vi "SERIAL_GetAngle.vi"(11 "navX DevRef":T1={"SerialPortRef"={"DevStatus"={"status"=FALSE, "code"=0, "source"=""}, "Serial Port Name"=""}, "Board Information"={"WhoAmI (50 | 0x32)"=0, "Board Revision"=0, "Firmware Major Version"=0, "Firmware Minor Version"=0, "NAVX_BOARD_CAPABILITY"={"OMNIMOUNT"=FALSE, "YAW_RESET"=FALSE, "VEL_AND_DISP"=FALSE}, "NAVX_BOARD_YAW_AXIS"={"BOARD_YAW_AXIS_UP"=FALSE, "BOARD_YAW_AXIS"=0}}, "Status"={"Update Rate Hz"=0, "Accelerometer Full-Scale Range"=0, "Gyro Full-Scale Range"=0, "NAVX_OP_STATUS"=0, "NAVX_CAL_STATUS"=0, "NAVX_SELFTEST_STATUS"=0, "NAVX_SENSOR_STATUS"={"MOVING"=FALSE, "YAW_STABLE"=FALSE, "MAG_DISTURBANCE"=FALSE, "ALTITUDE_VALID"=FALSE, "SEALEVEL_PRESS_SET"=FALSE, "FUSED_HEADING_VALID"=FALSE}}, "Offsets"={"Yaw"=50.0, "Quat W"=0.0, "Quat X"=0.0, "Quat Y"=0.0, "Quat Z"=0.0}, "Update Rate (4Hz-60Hz)"=50, "Nav6Mode (YPR)"=enum."RawSensorData", "refnum name"="", "error"={"status"=FALSE, "code"=0, "source"=""}, "Loop VI Refnum"=refnum, "Serial Port"=enum."Onboard RS-232"} {"Status"."NAVX_OP_STATUS" items=["INITIALIZING", "SELFTEST_IN_PROGRESS", "ERROR", "IMU_AUTOCAL_IN_PROGRESS", "NORMAL"]; "Status"."NAVX_CAL_STATUS" items=["IMU_CAL_STATE_MASK"=3, "IMU_CAL_INPROGRESS"=0, "IMU_CAL_ACCUMULATE"=1, "IMU_CAL_COMPLETE"=2, "MAG_CAL_COMPLETE"=4, "BARO_CAL_COMPLETE"=8]}) -> (1 "Valid?":bool, 2 "ContinuousAngle":dbl, 3 "navX DevRef 2":T1={"SerialPortRef"={"DevStatus"={"status"=FALSE, "code"=0, "source"=""}, "Serial Port Name"=""}, "Board Information"={"WhoAmI (50 | 0x32)"=0, "Board Revision"=0, "Firmware Major Version"=0, "Firmware Minor Version"=0, "NAVX_BOARD_CAPABILITY"={"OMNIMOUNT"=FALSE, "YAW_RESET"=FALSE, "VEL_AND_DISP"=FALSE}, "NAVX_BOARD_YAW_AXIS"={"BOARD_YAW_AXIS_UP"=FALSE, "BOARD_YAW_AXIS"=0}}, "Status"={"Update Rate Hz"=0, "Accelerometer Full-Scale Range"=0, "Gyro Full-Scale Range"=0, "NAVX_OP_STATUS"=0, "NAVX_CAL_STATUS"=0, "NAVX_SELFTEST_STATUS"=0, "NAVX_SENSOR_STATUS"={"MOVING"=FALSE, "YAW_STABLE"=FALSE, "MAG_DISTURBANCE"=FALSE, "ALTITUDE_VALID"=FALSE, "SEALEVEL_PRESS_SET"=FALSE, "FUSED_HEADING_VALID"=FALSE}}, "Offsets"={"Yaw"=50.0, "Quat W"=0.0, "Quat X"=0.0, "Quat Y"=0.0, "Quat Z"=0.0}, "Update Rate (4Hz-60Hz)"=50, "Nav6Mode (YPR)"=enum."RawSensorData", "refnum name"="", "error"={"status"=FALSE, "code"=0, "source"=""}, "Loop VI Refnum"=refnum, "Serial Port"=enum."Onboard RS-232"} {"Status"."NAVX_OP_STATUS" items=["INITIALIZING", "SELFTEST_IN_PROGRESS", "ERROR", "IMU_AUTOCAL_IN_PROGRESS", "NORMAL"]; "Status"."NAVX_CAL_STATUS" items=["IMU_CAL_STATE_MASK"=3, "IMU_CAL_INPROGRESS"=0, "IMU_CAL_ACCUMULATE"=1, "IMU_CAL_COMPLETE"=2, "MAG_CAL_COMPLETE"=4, "BARO_CAL_COMPLETE"=8]})   [LabVIEW 2014, in "navX-MXP IMU.lvlib"]
doc: "Returns the angle, in degrees, from the original heading that the robot is currently facing.\n\nNote that this angle is continuous (meaning that it can return values greater than 360 degrees and less than -360 degrees. You can device by 360 and use the remainder to yield and angle with a value from -360 to 360 degrees.\n\nThis VI is created to provide an interface which is compatible with the WPI LabVIEW Library GetAngle.vi ."
uses:
  navX-MXP IMU.lvlib
  TypeDefs/navX Serial DevRef.ctl
  <vilib>/Rock Robotics/WPI/SerialPort/WPI_SerialPortRef.ctl
  COMMON/TypeDefs/Data TypeDefs/navX Board Information.ctl
  COMMON/TypeDefs/Value TypeDefs/navX NAVX_BOARD_CAPABILITY.ctl
  COMMON/TypeDefs/Value TypeDefs/navX NAVX_BOARD_YAW_AXIS.ctl
  COMMON/TypeDefs/Data TypeDefs/navX Status Data.ctl
  COMMON/TypeDefs/Value TypeDefs/navX NAVX_OP_STATUS.ctl
  COMMON/TypeDefs/Value TypeDefs/navX NAVX_CAL_STATUS.ctl
  COMMON/TypeDefs/Value TypeDefs/navX NAVX_SENSOR_STATUS.ctl
  TypeDefs/navX Serial Mode.ctl
  IO/NI WPI/WPI_SerialPort_USB.ctl
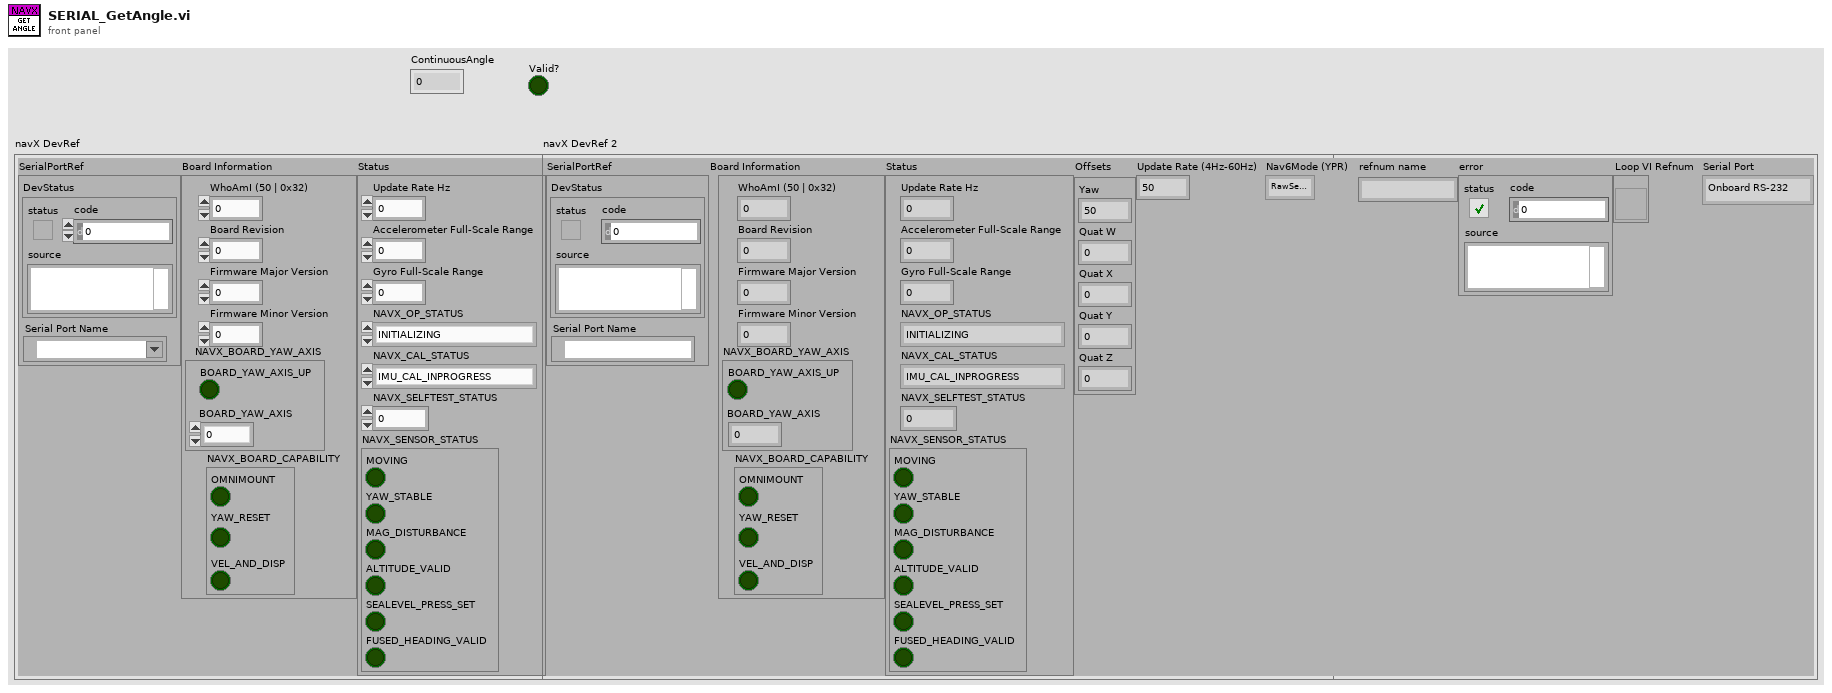
[diagram p1: front panel]
types:
  T1 = typedef "navX-MXP IMU.lvlib/navX Serial DevRef.ctl" = cluster{"SerialPortRef":T2, "Board Information":T3, "Status":T6, "Offsets":cluster{"Yaw":dbl, "Quat W":dbl, "Quat X":dbl, "Quat Y":dbl, "Quat Z":dbl}, "Update Rate (4Hz-60Hz)":u8, "Nav6Mode (YPR)":T10, "refnum name":string, "error":errorcluster, "Loop VI Refnum":refnum<vi>, "Serial Port":T11}
  T2 = typedef "WPI_SerialPortRef.ctl" = cluster{"DevStatus":errorcluster, "Serial Port Name":refnum<visa-resource-name>}
  T3 = typedef "navX-MXP IMU.lvlib/navX Board Information.ctl" = cluster{"WhoAmI (50 | 0x32)":u8, "Board Revision":u8, "Firmware Major Version":u8, "Firmware Minor Version":u8, "NAVX_BOARD_CAPABILITY":T4, "NAVX_BOARD_YAW_AXIS":T5}
  T4 = typedef "navX-MXP IMU.lvlib/navX NAVX_BOARD_CAPABILITY.ctl" = cluster{"OMNIMOUNT":bool, "YAW_RESET":bool, "VEL_AND_DISP":bool}
  T5 = typedef "navX-MXP IMU.lvlib/navX NAVX_BOARD_YAW_AXIS.ctl" = cluster{"BOARD_YAW_AXIS_UP":bool, "BOARD_YAW_AXIS":u8}
  T6 = typedef "navX-MXP IMU.lvlib/navX Status Data.ctl" = cluster{"Update Rate Hz":u8, "Accelerometer Full-Scale Range":u8, "Gyro Full-Scale Range":u16, "NAVX_OP_STATUS":T7, "NAVX_CAL_STATUS":T8, "NAVX_SELFTEST_STATUS":u8, "NAVX_SENSOR_STATUS":T9}
  T7 = typedef "navX-MXP IMU.lvlib/navX NAVX_OP_STATUS.ctl" = u8
  T8 = typedef "navX-MXP IMU.lvlib/navX NAVX_CAL_STATUS.ctl" = u8
  T9 = typedef "navX-MXP IMU.lvlib/navX NAVX_SENSOR_STATUS.ctl" = cluster{"MOVING":bool, "YAW_STABLE":bool, "MAG_DISTURBANCE":bool, "ALTITUDE_VALID":bool, "SEALEVEL_PRESS_SET":bool, "FUSED_HEADING_VALID":bool}
  T10 = typedef "navX-MXP IMU.lvlib/navX Serial Mode.ctl" = enum16{"RawSensorData", "ProcessedData"}
  T11 = typedef "navX-MXP IMU.lvlib/WPI_SerialPort_USB.ctl" = enum16{"Onboard RS-232", "MXP TTL", "USB"}
  T12 = typedef "navX-MXP IMU.lvlib/navX YPRH Data.ctl" = cluster{"Yaw":dbl, "Pitch":dbl, "Roll":dbl, "Heading":dbl}
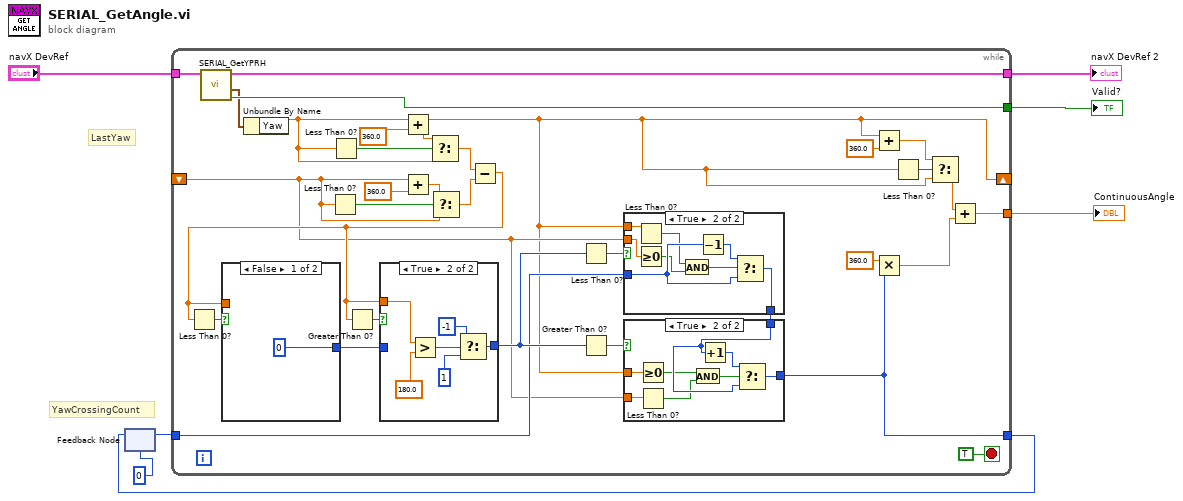
[diagram p0: block diagram]
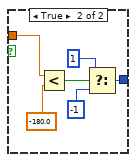
[diagram p5: hidden frame]
diagram:
  # "YawCrossingCount"
  # "LastYaw"
  n1 = feedback #1(0) -> (w3:i32)
  n2 = while {
    shift-right: [w10] -> _
    shift-left: _ -> [w11]
    tunnel: [w38] -> w5
    tunnel: "navX DevRef" -> [w8]
    tunnel: [w35] -> w6
    tunnel: [w25] -> w4
    tunnel: w3 -> [w23]
    tunnel: [w22] -> w1
    stop <- TRUE stop-if-true
    n3 = call "SERIAL_GetYPRH.vi"("navX Ref Object"=w8) -> ("Valid"=w38:bool, "YPRH"=w34:T12, "navX Ref Object"=w35:T1)  [unwired: 8 in]
    n4 = Unbundle By Name(w34) -> ("Yaw"=w10:dbl)
    n5 = Less Than 0?(x=w11) -> (x < 0?=w15:bool)
    n6 = Less Than 0?(x=w10) -> (x < 0?=w16:bool)
    n7 = Add(x=w10, y=360.0) -> (x+y=w9:dbl)
    n8 = Add(x=w11, y=360.0) -> (x+y=w12:dbl)
    n9 = Select(t=w9, s=w16, f=w10) -> (s? t:f=w14:dbl)
    n10 = Select(t=w12, s=w15, f=w11) -> (s? t:f=w13:dbl)
    n11 = Subtract(x=w14, y=w13) -> (x-y=w17:dbl)
    n12 = Less Than 0?(x=w17) -> (x < 0?=w19:bool)
    n13 = case shown="False" w19 {
      tunnel: [0 w67] -> w33
      tunnel: w17 -> [_ w66]
      frame False {
      }
      frame True {
        n14 = Less?(x=w66, y=-180.0) -> (x < y?=w70:bool)
        n15 = Select(t=1, s=w70, f=-1) -> (s? t:f=w67:i32)
      }
    }
    n16 = Greater Than 0?(x=w17) -> (x > 0?=w18:bool)
    n17 = case shown="True" w18 {
      tunnel: [w58 w60] -> w30
      tunnel: w33 -> [w58 _]
      tunnel: w17 -> [_ w59]
      frame False {
      }
      frame True {
        n18 = Greater?(x=w59, y=180.0) -> (0:w63:bool)
        n19 = Select(t=-1, s=w63, f=1) -> (s? t:f=w60:i32)
      }
    }
    n20 = Less Than 0?(x=w30) -> (x < 0?=w32:bool)
    n21 = Greater Than 0?(x=w30) -> (x > 0?=w31:bool)
    n22 = case shown="True" w32 {
      tunnel: w23 -> [w49 w56]
      tunnel: w10 -> [_ w54]
      tunnel: [w49 w55] -> w24
      tunnel: w11 -> [_ w53]
      frame False {
      }
      frame True {
        n23 = Less Than 0?(x=w54) -> (x < 0?=w52:bool)
        n24 = Greater Or Equal To 0?(x=w53) -> (x >= 0?=w51:bool)
        n25 = And(x=w52, y=w51) -> (x .and. y?=w50:bool)
        n26 = Decrement(x=w56) -> (x-1=w57:i32)
        n27 = Select(t=w57, s=w50, f=w56) -> (s? t:f=w55:i32)
      }
    }
    n28 = case shown="True" w31 {
      tunnel: w10 -> [_ w45]
      tunnel: w24 -> [w40 w47]
      tunnel: [w40 w46] -> w22
      tunnel: w11 -> [_ w44]
      frame False {
      }
      frame True {
        n29 = Greater Or Equal To 0?(x=w45) -> (x >= 0?=w42:bool)
        n30 = Less Than 0?(x=w44) -> (x < 0?=w41:bool)
        n31 = And(x=w42, y=w41) -> (x .and. y?=w43:bool)
        n32 = Increment(x=w47) -> (x+1=w48:i32)
        n33 = Select(t=w48, s=w43, f=w47) -> (s? t:f=w46:i32)
      }
    }
    n34 = Add(x=w10, y=360.0) -> (x+y=w20:dbl)
    n35 = Multiply(x=360.0, y=w22) -> (x*y=w26:dbl)
    n36 = Less Than 0?(x=w10) -> (x < 0?=w29:bool)
    n37 = Select(t=w20, s=w29, f=w10) -> (s? t:f=w28:dbl)
    n38 = Add(x=w28, y=w26) -> (x+y=w25:dbl)
  }
  "Valid?" <- w5
  "navX DevRef 2" <- w6
  "ContinuousAngle" <- w4
  n39 = feedback-in #1(w1) -> ()
